vi "_TEST.vi"() -> ()   [LabVIEW 2019, in "lv-apt-json-file.lvlib"]
uses:
  lv-apt-json-file.lvlib
  cb48201e-b36a-4d73-bd5e-d1f1185de09b.vi
  3ec21194-c1e0-4b26-99b6-e5851eab70d9.vi
  28cda003-a995-4c9f-9592-8600d2dd0259.vi
  69f0ba20-7e38-4809-9103-35991914e280.vi
  <vilib>/Utility/error.llb/Clear Errors.vi
  Remove Comments.vi
  cb48201e-b36a-4d73-bd5e-d1f1185de09b.vi/56b3740c-bc24-458e-95d3-5fd248b79467.vi
  3ec21194-c1e0-4b26-99b6-e5851eab70d9.vi/d798efcf-5860-43f0-a975-5f218ec3e1d9.vi
  28cda003-a995-4c9f-9592-8600d2dd0259.vi/9a2716c5-0d63-480a-b6df-be1f45c7617f.vi
  69f0ba20-7e38-4809-9103-35991914e280.vi/4ac13cff-22b6-4e4f-88b1-0c860d13e2f0.vi
  <userlib>/NEVSTOP-Programming-Palette/Configuration/Ini/TextToLines.vi
  <userlib>/_OpenG.lib/array/array.llb/Filter 1D Array__ogtk.vi
  <userlib>/_OpenG.lib/array/array.llb/Filter 1D Array (U8)__ogtk.vi
  <userlib>/NEVSTOP-Programming-Palette/Configuration/Ini/LinesToText.vi
  <vilib>/Utility/error.llb/Error Cluster From Error Code.vi
  <userlib>/_OpenG.lib/lvdata/lvdata.llb/Get TDEnum from Data__ogtk.vi
  IsAttrMap.vi
  <userlib>/_OpenG.lib/string/string.llb/Format Variant Into String__ogtk.vi
  <vilib>/addons/_JKI.lib/Serialization/JSON/JKI JSON Serialization.lvlib
panel:
  out "Cluster 4":variant=variant(cluster{"STR":string, "CLUSTER2":cluster{"STR":string, "BOOLEAN":bool, "enum":enum16{"a", "b", "c"}}, "FALSE":bool} {"STR"="CLUSTER->STR", "CLUSTER2"={"STR"="CLUSTER2->STR", "BOOLEAN"=TRUE, "enum"=enum."a"}, "FALSE"=FALSE})
  out "appended array":variant[](array[variant])
  out "AttrMap 2":variant=variant("CLUSTER2"=variant("BOOLEAN"=variant(bool TRUE), "STR"=variant(string "abv"), "enum"=variant(enum16{"a", "b", "c"} enum."a")), "FALSE"=variant(bool FALSE), "STR"=variant(string "CLUSTER->STR"))
  out "AttrMap":variant=variant("CLUSTER2"=variant("FALSE"=variant(bool FALSE), "STR"=variant(string "abv"), "abde"=variant(string "asdf")), "STR"=variant(string "CLUSTER->STR"))
  out "Json":string="{\r\n    \"FALSE\":false,\r\n    \"STR\":\"CLUSTER->STR\",\r\n    \"CLUSTER2\":{\r\n        \"BOOLEAN\":true,\r\n        \"STR\":\"CLUSTER2->STR\",\r\n        \"enum\":\"a\"\r\n    }\r\n}"
  out "error out 2":errorcluster
  out "error out":errorcluster
  out "Cluster 3":variant=variant(cluster{"STR":string, "CLUSTER2":cluster{"STR":string, "BOOLEAN":bool, "enum":enum16{"a", "b", "c"}}, "FALSE":bool} {"STR"="CLUSTER->STR", "CLUSTER2"={"STR"="abv", "BOOLEAN"=TRUE, "enum"=enum."a"}, "FALSE"=FALSE})
  out "Cluster 2":variant=variant(cluster{"STR":string, "CLUSTER2":cluster{"STR":string, "BOOLEAN":bool, "enum":enum16{"a", "b", "c"}}, "FALSE":bool} {"STR"="CLUSTER->STR", "CLUSTER2"={"STR"="abv", "BOOLEAN"=TRUE, "enum"=enum."a"}, "FALSE"=FALSE})
  in  "JSON String 2":string="{\r\n    \"STR\":\"CLUSTER->STR\",\r\n    \"CLUSTER2\":{\r\n        \"FALSE\":false,\r\n        \"STR\":\"abv\"\r\n    },\n\"abde\":\"asdf\"\r\n}"
  out "JSON String":string="{\r\n    \"STR\":\"CLUSTER->STR\",\r\n    \"CLUSTER2\":{\r\n        \"STR\":\"CLUSTER2->STR\",\r\n        \"BOOLEAN\":true,\r\n        \"enum\":\"a\"\r\n    },\r\n    \"FALSE\":false\r\n}"
  out "Cluster":variant=variant(cluster{"STR":string, "CLUSTER2":cluster{"STR":string, "BOOLEAN":bool, "enum":enum16{"a", "b", "c"}}, "FALSE":bool} {"STR"="CLUSTER->STR", "CLUSTER2"={"STR"="CLUSTER2->STR", "BOOLEAN"=TRUE, "enum"=enum."a"}, "FALSE"=FALSE})
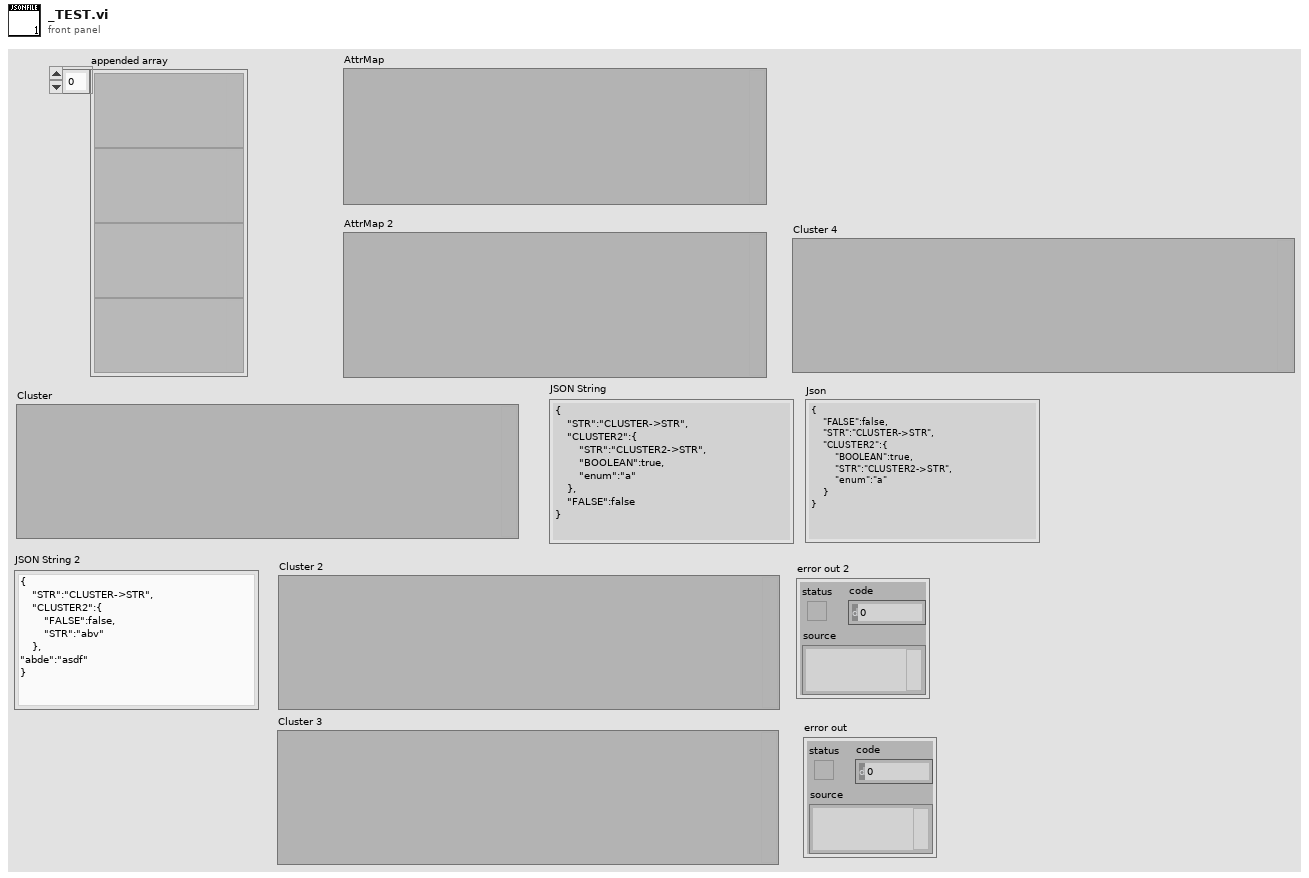
[diagram p1: front panel]
types:
  T1 = cluster{"STR":string, "CLUSTER2":cluster{"STR":string, "BOOLEAN":bool, "enum":enum16{"a", "b", "c"}}, "FALSE":bool}
  T2 = typedef "lv-apt-json-file.lvlib/Def-AttrMap.ctl" = variant
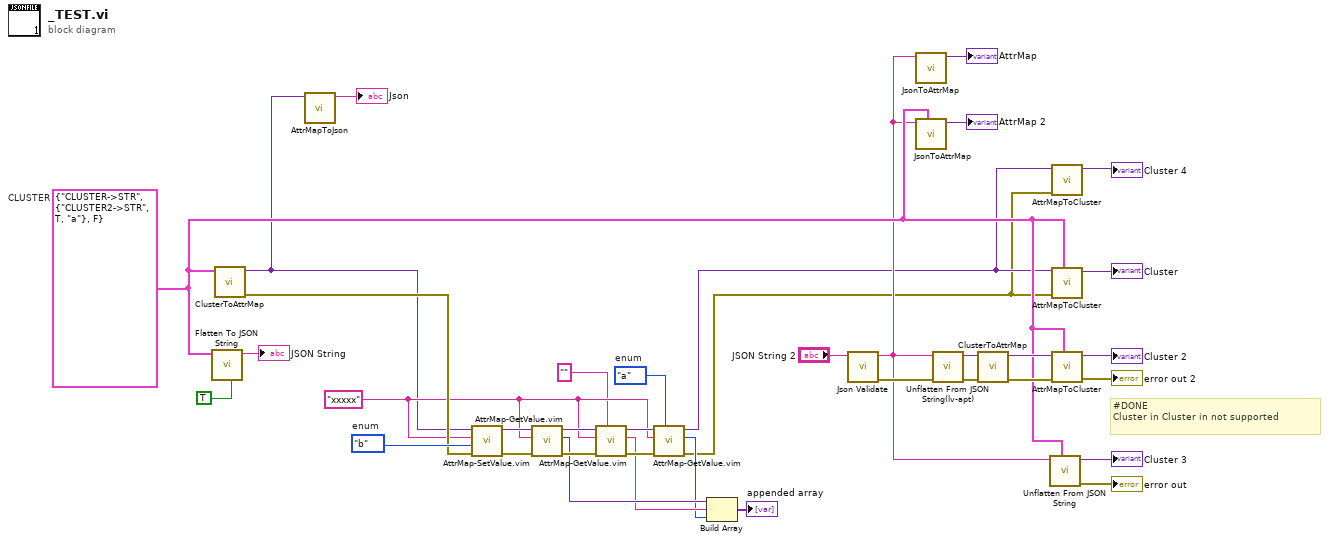
[diagram p0: block diagram]
diagram:
  w13 = enum16{"a", "b", "c"}."a"  # enum
  w17 = enum16{"a", "b", "c"}."b"  # enum
  w12 = "xxxxx" ("Key(String/Enum)")
  w21 = T1 {"STR"="CLUSTER->STR", "CLUSTER2"={"STR"="CLUSTER2->STR", "BOOLEAN"=TRUE, "enum"=enum."a"}, "FALSE"=FALSE}  # CLUSTER
  # "#DONE\nCluster in Cluster in not supported"
  n1 = call <vilib>:"Flatten To JSON String.vi"("Enums As String (F)"=TRUE, "Variant"=w21) -> ("JSON String"=→"JSON String":string)  [unwired: 8 in, 1 out]
  n2 = call "ClusterToAttrMap.vi"("data"=w21) -> ("error out"=w16:errorcluster, "AttrMap"=w4:T2)  [unwired: 9 in]
  n3 = call "AttrMapToJson.vi"("AttrMap"=w4) -> ("Json"=→"Json":string)  [unwired: 9 in, 1 out]
  n4 = call "AttrMap-SetValue.vim"("error in (no error)"=w16, "Value"=w17, "Key(String/Enum)"=w12, "AttrMap in"=w4) -> ("error out"=w18:errorcluster, "AttrMap out"=w19:T2)  [unwired: 6 in]
  n5 = call "AttrMap-GetValue.vim"("error in (no error)"=w18, "Key(String/Enum)"=w12, "AttrMap in"=w19) -> ("error out"=w10:errorcluster, "Value"=w8:variant, "AttrMap out"=w15:variant)  [unwired: 5 in, 1 out]
  n6 = call "AttrMap-GetValue.vim"("Type"="" ("Key(String/Enum)"), "error in (no error)"=w10, "Key(String/Enum)"=w12, "AttrMap in"=w15) -> ("error out"=w9:errorcluster, "Value"=w7:string, "AttrMap out"=w14:variant)  [unwired: 4 in, 1 out]
  n7 = call "AttrMap-GetValue.vim"("Type"=w13, "error in (no error)"=w9, "Key(String/Enum)"=w12, "AttrMap in"=w14) -> ("error out"=w2:errorcluster, "Value"=w6:enum16{"a", "b", "c"}, "AttrMap out"=w3:variant)  [unwired: 4 in, 1 out]
  n8 = Build Array(w8, w7, w6) -> (→"appended array":variant[])
  n9 = call "Json Validate.vi"("String"="JSON String 2") -> ("error out"=w29:errorcluster, "Json without comments"=w20:string)  [unwired: 7 in, 2 out]
  n10 = call "JsonToAttrMap.vi"("Json"=w20) -> ("AttrMap"=→"AttrMap":T2)  [unwired: 9 in, 1 out]
  n11 = call "JsonToAttrMap.vi"("Type and Defaults"=w21, "Json"=w20) -> ("AttrMap"=→"AttrMap 2":T2)  [unwired: 8 in, 1 out]
  n12 = call "Unflatten From JSON String(lv-apt).vi"("error in (no error)"=w29, "JSON String"=w20) -> ("error out"=w34:errorcluster, "Variant"=w35:variant)  [unwired: 8 in]
  n13 = call "ClusterToAttrMap.vi"("error in (no error)"=w34, "data"=w35) -> ("error out"=w32:errorcluster, "AttrMap"=w33:T2)  [unwired: 8 in]
  n14 = call <vilib>:"Unflatten From JSON String.vi"("Type and Defaults"=w21, "JSON String"=w20) -> ("error out"=→"error out":errorcluster, "Variant"=→"Cluster 3":variant)  [unwired: 8 in]
  n15 = call "AttrMapToCluster.vi"("error in (no error)"=w2, "AttrMap"=w3) -> ("Cluster"=→"Cluster 4":variant)  [unwired: 8 in, 1 out]
  n16 = call "AttrMapToCluster.vi"("Prototype"=w21, "error in (no error)"=w2, "AttrMap"=w3) -> ("Cluster"=→"Cluster":variant)  [unwired: 7 in, 1 out]
  n17 = call "AttrMapToCluster.vi"("Prototype"=w21, "error in (no error)"=w32, "AttrMap"=w33) -> ("error out"=→"error out 2":errorcluster, "Cluster"=→"Cluster 2":variant)  [unwired: 7 in]
